vi "Find XML Paths to Edit.vi"(8 "error in":errorcluster, 11 "consumer data":T1) -> (0 "error out":errorcluster, 1 "engine path":string, 2 "cd install directory":string, 3 "consumer data out":T1)   [LabVIEW 2020, in "Template Tool.lvlib"]
uses:
  Template Tool.lvlib
  Consumer Data.ctl
  Project Build Specs.ctl
  <vilib>/regexp/Match Regular Expression.xnode
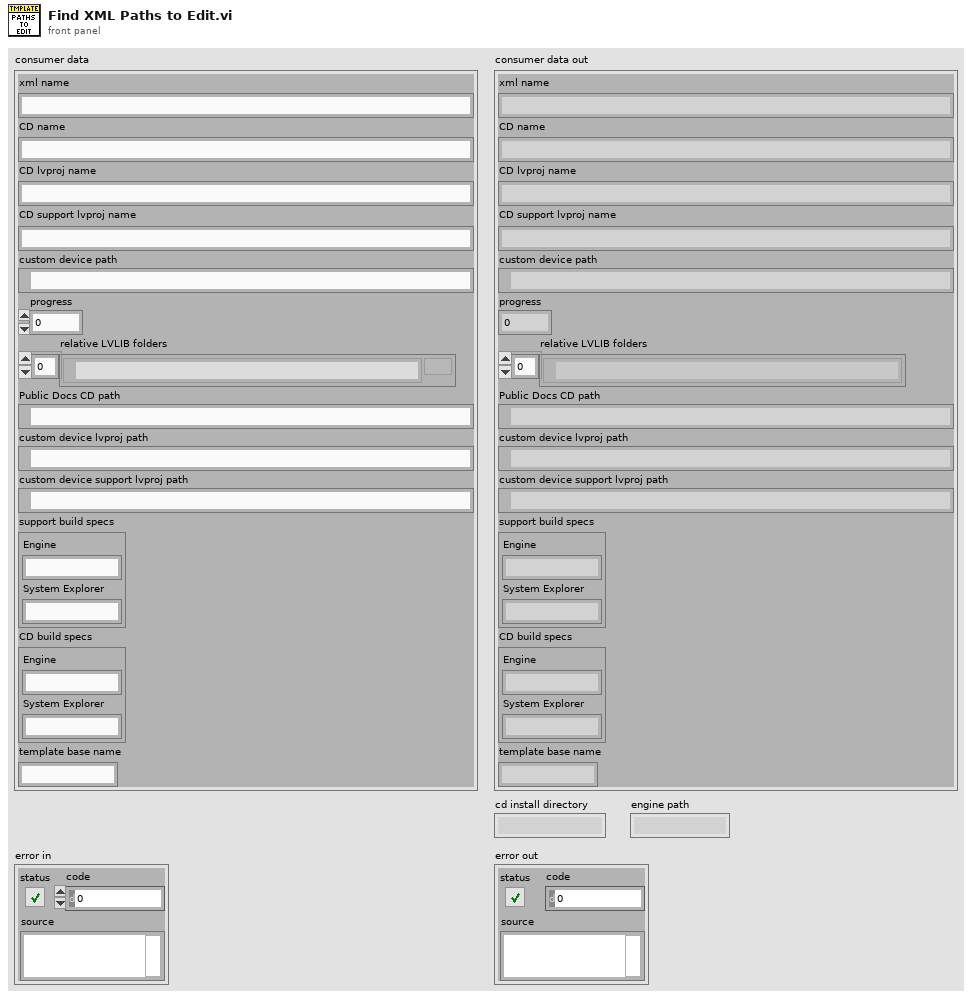
[diagram p1: front panel]
types:
  T1 = typedef "Template Tool.lvlib/Consumer Data.ctl" = cluster{"xml name":string, "CD name":string, "CD lvproj name":string, "CD support lvproj name":string, "custom device path":path, "progress":u8, "relative LVLIB folders":path[], "Public Docs CD path":path, "custom device lvproj path":path, "custom device support lvproj path":path, "support build specs":T2, "CD build specs":T2, "template base name":string}
  T2 = typedef "Template Tool.lvlib/Project Build Specs.ctl" = cluster{"Engine":string, "System Explorer":string}
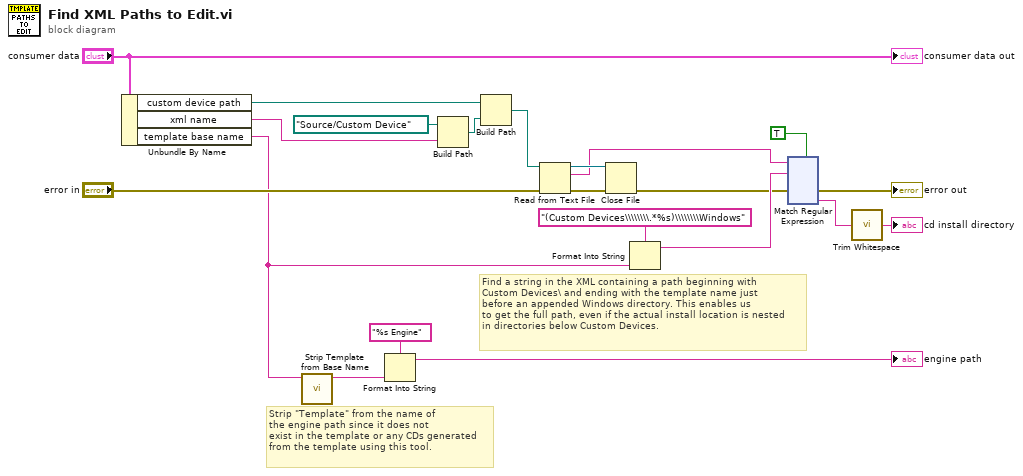
[diagram p0: block diagram]
diagram:
  # "Strip \"Template\" from the name of\nthe engine path since it does not\nexist in the template or any CDs generated\nfrom the template using this tool."
  # "Find a string in the XML containing a path beginning with\nCustom Devices\\ and ending with the template name just\nbefore an appended Windows directory. This enables us\nto get the full path, even if the actual install location is nested\nin directories below Custom Devices."
  n1 = Unbundle By Name("consumer data") -> ("custom device path"=w8:path, "xml name"=w6:string, "template base name"=w2:string)
  n2 = call "Strip Template from Base Name.vi"("template base name"=w2) -> ("stripped base name"=w1:string)  [unwired: 9 in, 1 out]
  n3 = Format Into String(format string="%s Engine", w1) -> (resulting string=→"engine path":string)  [unwired: 2 in, 1 out]
  n4 = Build Path(base path=path "Source/Custom Device", name or relative path=w6) -> (appended path=w5:path)
  n5 = Build Path(base path=w8, name or relative path=w5) -> (appended path=w21:path)
  n6 = Read from Text File(file (use dialog)=w21, error in="error in") -> (refnum out=w18:refnum<file>, text=w14:string, error out=w19:errorcluster)  [unwired: 2 in, 1 out]
  n7 = Close File(refnum=w18, error in=w19) -> (error out=w11:errorcluster)  [unwired: 1 out]
  n8 = Format Into String(format string="(Custom Devices\\\\\\\\.*%s)\\\\\\\\Windows" ("search string"), w2) -> (resulting string=w15:string)  [unwired: 2 in, 1 out]
  n9 = xnode "Match Regular Expression"("input string"=w14, "regular expression"=w15, "error in"=w11, "multiline? (F)"=TRUE) -> ("error out"=→"error out":errorcluster, "submatch 1"=w13:string)  [unwired: 2 in, 4 out]
  n10 = call <vilib>:"Trim Whitespace.vi"("string"=w13) -> ("trimmed string"=→"cd install directory":string)  [unwired: 1 in]
  "consumer data out" <- "consumer data"
